vi "Read & Write Configuration OO-DB.vi"() -> ()   [LabVIEW 2012, in "DB-Configuration.lvlib"]
doc: "Read object oriented configuration data from database using the configuration class.\n\nLizenziert unter EUPL V. 1.1"
uses:
  Configuration/Classes/Configuration/Configuration.lvclass
  ODBC-Interface/ODBC-Interface.lvclass
  Introduction/Examples/Classes/Section 1/Section 1.lvclass
  DB-Configuration.lvlib
  Configuration/Classes/Section/Section.lvclass
panel:
  in  "password":string
  in  "userID":string="postgres"
  in  "connection information":string="PostgreSQL30"
  out "Sections":T1(array[cluster])
  out "Configuration out":refnum<class "Configuration.lvclass">
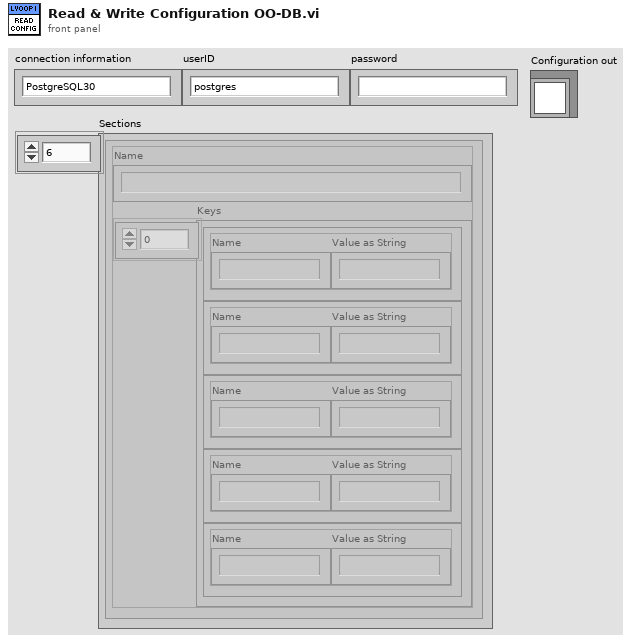
[diagram p1: front panel]
types:
  T1 = cluster{"Name":string, "Keys":cluster{"Name":string, "Value as String":string}[]}[]
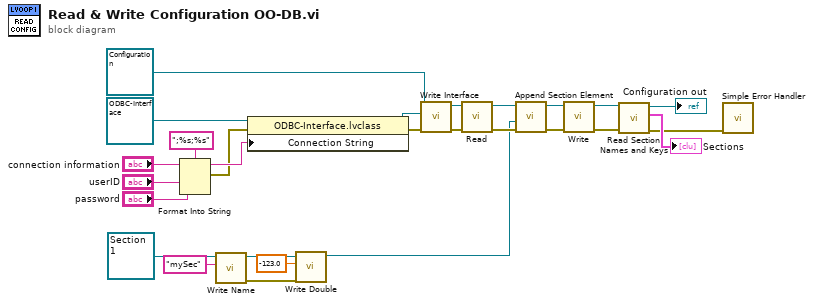
[diagram p0: block diagram]
diagram:
  n1 = Format Into String(format string=";%s;%s", initial string="connection information", "userID", "password") -> (resulting string=w14:string, error out=w13:errorcluster)  [unwired: 1 in]
  n2 = call "Write Name.vi"("Name"="mySec", "Section in"=refnum<class "Section 1.lvclass"> refnum ("LVOOP Introduction.lvlib:Section 1.lvclass")) -> ("error out"=w8:errorcluster, "Section out"=w10:refnum<class "Section 1.lvclass">)  [unwired: 8 in]
  n3 = property class="ODBC-Interface.lvclass"(reference=refnum<class "ODBC-Interface.lvclass"> refnum ("DB-Configuration.lvlib:ODBC-Interface.lvclass"), error in=w13, "Connection String"=w14) -> (reference out=w23:refnum<class "ODBC-Interface.lvclass">, error out=w26:errorcluster)
  n4 = call "Write Double.vi"("error in (no error)"=w8, "Double"=-123.0, "Section 1 in"=w10) -> ("Section 1 out"=w1:refnum<class "Section 1.lvclass">)  [unwired: 7 in, 1 out]
  n5 = call "Write Interface.vi"("error in (no error)"=w26, "Interface"=w23, "Configuration in"=refnum<class "Configuration.lvclass"> refnum) -> ("error out"=w25:errorcluster, "Configuration out"=w24:refnum<class "Configuration.lvclass">)  [unwired: 7 in]
  n6 = call "Read.vi"("error in (no error)"=w25, "Configuration"=w24) -> ("error out"=w4:errorcluster, "Configuration out"=w5:refnum<class "Configuration.lvclass">)  [unwired: 8 in]
  n7 = call "Append Section Element.vi"("error in (no error)"=w4, "Section"=w1, "Configuration in"=w5) -> ("error out"=w7:errorcluster, "Configuration out"=w6:refnum<class "Configuration.lvclass">)  [unwired: 7 in]
  n8 = call "Write.vi"("error in (no error)"=w7, "Configuration in"=w6) -> ("error out"=w2:errorcluster, "Configuration out"=w3:refnum<class "Configuration.lvclass">)  [unwired: 8 in]
  n9 = call "Read Section Names and Keys.vi"("error in (no error)"=w2, "Configuration in"=w3) -> ("error out"=w21:errorcluster, "Sections"=→"Sections":T1, "Configuration out"=→"Configuration out":refnum<class "Configuration.lvclass">)  [unwired: 7 in]
  n10 = call <vilib>:"Simple Error Handler.vi"("error in (no error)"=w21) -> ()  [unwired: 4 in, 5 out]
